vi "AutoSteerAngle_rev0.vi"(6 "CurrentDirection":dbl, 8 "Ycurrent":dbl, 9 "Xcurrent":dbl, 10 "Ywaypoint":dbl, 11 "Xwaypoint":dbl) -> (2 "SteerAngle":dbl)   [LabVIEW 2010]
doc: "This VI calculates steering angle from current robot position to next waypoint."
uses:
  <vilib>/addons/control/pid/pid.llb/PID (DBL).vi
  <vilib>/addons/control/pid/NI_PID_pid.lvlib
panel:
  out "Waveform Chart 2":dbl(graph)
  out "output range":cluster{"output high":dbl, "output low":dbl}={"output high"=100.0, "output low"=-100.0} {"output low" format="%.2f"; "output high" format="%.2f"}
  in  "PID gains":T1={"proportional gain (Kc)"=20.0, "integral time (Ti, min)"=0.008, "derivative time (Td, min)"=0.001} {"derivative time (Td, min)" step=1e-05 format="%.5f"; "integral time (Ti, min)" step=0.0001 format="%.4f"; "proportional gain (Kc)" step=0.001 format="%.4f"}
  out "Waveform Chart":cluster{dbl, "CurrentDirection":dbl}(graph)
  out "towaypoint":dbl
  # "This Vi calculates sttering angle \nfrom current position to \nnext waypoint"
  # "0.5kts\n0.100\n0.0038\n0.00003"
  # "1.0kts\n0.087\n0.000\n0.0000"
  # "45\n-45"
  # "in degreees"
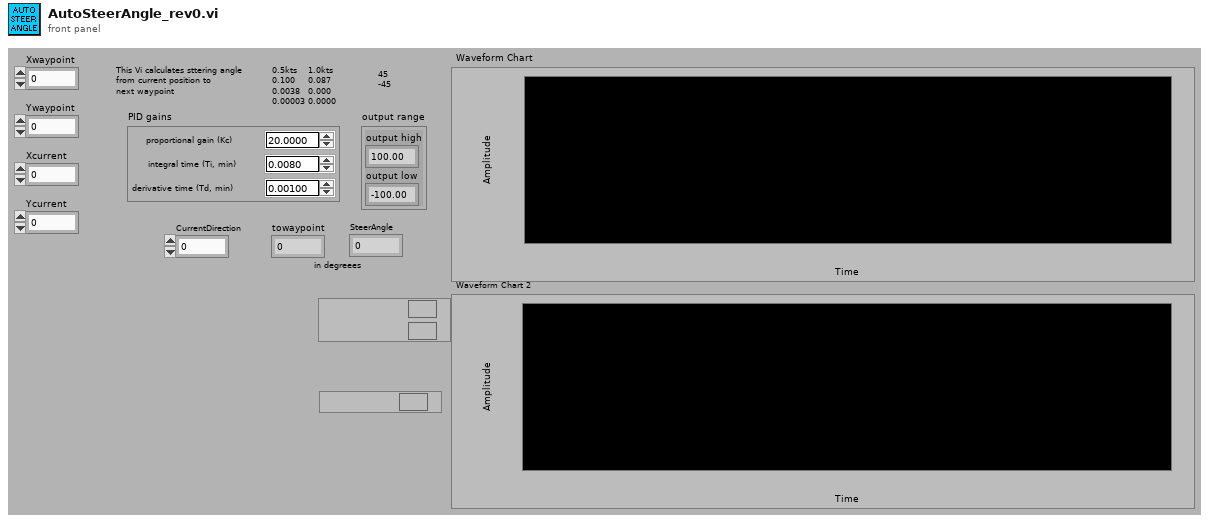
[diagram p1: front panel]
types:
  T1 = cluster{"proportional gain (Kc)":dbl, "integral time (Ti, min)":dbl, "derivative time (Td, min)":dbl}
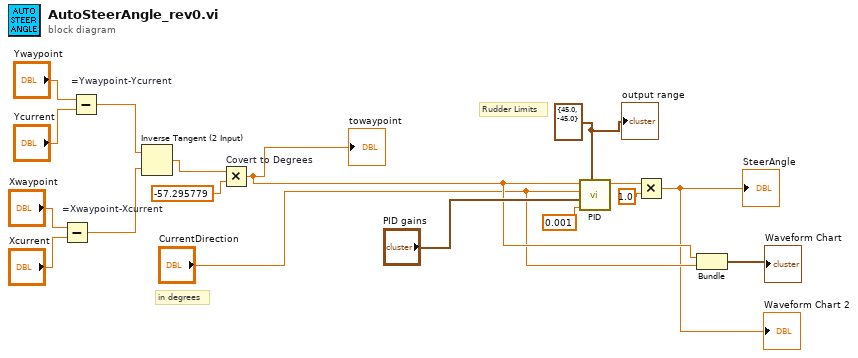
[diagram p0: block diagram]
diagram:
  w1 = cluster{"output high":dbl, "output low":dbl} {"output high"=45.0, "output low"=-45.0} ("output range")
  # "Rudder Limits"
  # "in degrees"
  n1 = Subtract "=Xwaypoint-Xcurrent"(x="Xwaypoint", y="Xcurrent") -> (x-y=w12:dbl)
  n2 = Subtract "=Ywaypoint-Ycurrent"(x="Ywaypoint", y="Ycurrent") -> (x-y=w13:dbl)
  n3 = Inverse Tangent (2 Input)(1:w12, 2:w13) -> (0:w10:dbl)
  n4 = Multiply "Covert to Degrees"(x=w10, y=-57.295779) -> (x*y=w5:dbl)
  "towaypoint" <- w5
  n5 = call-poly <vilib>:"PID.vi"("output range"=w1, "dt (s)"=0.001, "PID gains"="PID gains", "process variable"="CurrentDirection", "setpoint"=w5) -> ("output"=w7:dbl)  [unwired: 5 in, 1 out]
  n6 = Multiply(x=w7, y=1.0) -> (x*y=→"SteerAngle" →"Waveform Chart 2":dbl)
  n7 = Bundle(w5, "CurrentDirection"="CurrentDirection") -> (→"Waveform Chart":cluster{dbl, "CurrentDirection":dbl})  [unwired: 1 in]
  "output range" <- w1
